vi "Check for Game Winner.vi"(8 "error in":errorcluster, 11 "Array - Numeric":dbl[][](array[numeric])) -> (0 "error out":errorcluster, 1 "Tie Game":bool, 2 "Player 1 wins":bool, 3 "Game Won":bool)   [LabVIEW 2021]
panel:
  out "Player 2 wins":bool
  out "diag subarray 2":dbl[](array[numeric])
  out "diag subarray 1":dbl[](array[numeric])
  out "col subarray 1":dbl[](array[numeric])
  out "col subarray 2":dbl[](array[numeric])
  out "col subarray 3":dbl[](array[numeric])
  out "row subarray 3":dbl[](array[numeric])
  out "row subarray 2":dbl[](array[numeric])
  out "row subarray 1":dbl[](array[numeric])
  # "Check rows\nCheck columns\nCheck diagonal 1 (top left to bot right)\nCheck diagonal 2 (bot left to top right)"
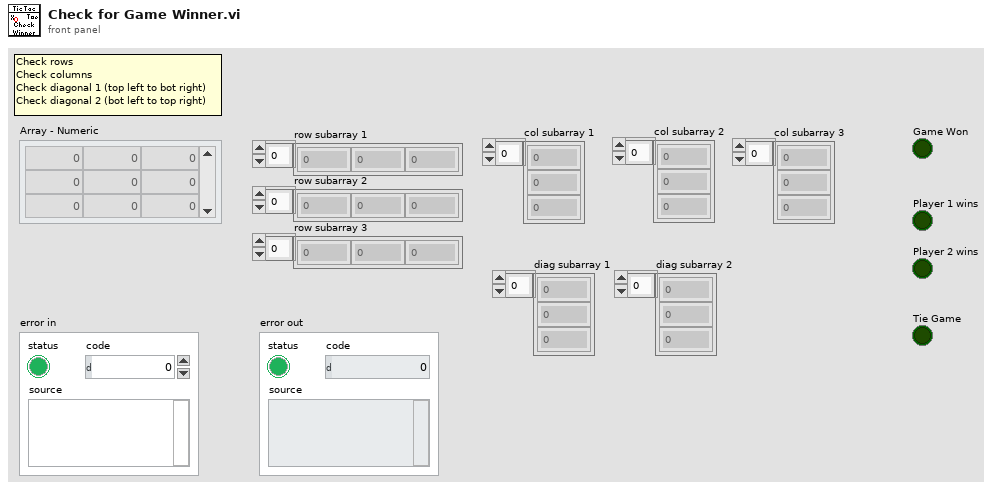
[diagram p1: front panel]
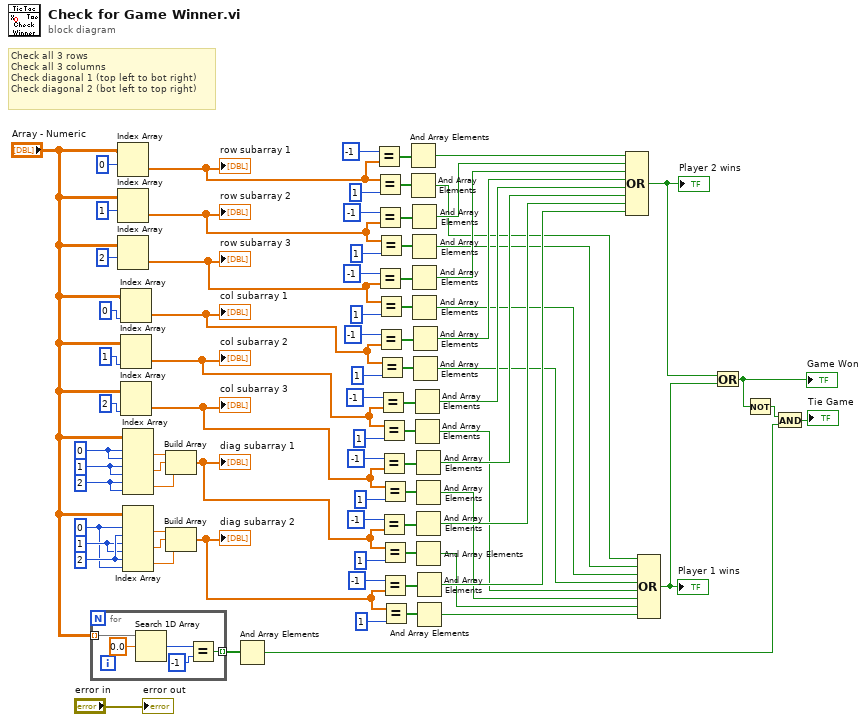
[diagram p0: block diagram]
diagram:
  w68 = 2 ("index (row)")
  w67 = 1 ("index (row)")
  w66 = 0 ("index (row)")
  w75 = 2 ("index (row)")
  w76 = 1 ("index (row)")
  w77 = 0 ("index (row)")
  # "Check all 3 rows\nCheck all 3 columns\nCheck diagonal 1 (top left to bot right)\nCheck diagonal 2 (bot left to top right)"
  n1 = for {
    tunnel: "Array - Numeric" -> [w88] mode=indexing
    tunnel: [w84] -> w5 mode=indexing
    n2 = Search 1D Array(1D array=w88, element=0.0) -> (index of element=w86:i32)  [unwired: 1 in]
    n3 = Equal?(x=w86, y=-1 ("index (row)")) -> (x = y?=w84:bool)
  }
  n4 = Index Array(array="Array - Numeric", index (row)=0) -> (element=w63:dbl[])  [unwired: 1 in]
  "row subarray 1" <- w63
  n5 = Index Array(array="Array - Numeric", index (row)=1) -> (element=w48:dbl[])  [unwired: 1 in]
  "row subarray 2" <- w48
  n6 = Index Array(array="Array - Numeric", index (row)=2) -> (element=w47:dbl[])  [unwired: 1 in]
  "row subarray 3" <- w47
  n7 = Index Array(array="Array - Numeric", index (col)=0 ("index (row)")) -> (element=w46:dbl[])  [unwired: 1 in]
  "col subarray 1" <- w46
  n8 = Index Array(array="Array - Numeric", index (col)=1 ("index (row)")) -> (element=w29:dbl[])  [unwired: 1 in]
  "col subarray 2" <- w29
  n9 = Index Array(array="Array - Numeric", index (col)=2 ("index (row)")) -> (element=w28:dbl[])  [unwired: 1 in]
  "col subarray 3" <- w28
  n10 = Index Array(array="Array - Numeric", index (row) #1=w77, index (col) #1=w77, index (row) #2=w76, index (col) #2=w76, index (row) #3=w75, index (col) #3=w75) -> (element #1=w74:dbl, element #2=w73:dbl, element #3=w72:dbl)
  n11 = Index Array(array="Array - Numeric", index (row) #1=w66, index (col) #1=w68, index (row) #2=w67, index (col) #2=w67, index (row) #3=w68, index (col) #3=w66) -> (element #1=w69:dbl, element #2=w70:dbl, element #3=w71:dbl)
  n12 = Build Array(w74, w73, w72) -> (w27:dbl[])
  "diag subarray 1" <- w27
  n13 = Build Array(w69, w70, w71) -> (w26:dbl[])
  "diag subarray 2" <- w26
  n14 = And Array Elements(Boolean array=w5) -> (logical AND=w2:bool)
  n15 = Equal?(x=-1 ("index (row)"), y=w63) -> (x = y?=w62:bool[])
  n16 = Equal?(x=w63, y=1 ("index (row)")) -> (x = y?=w61:bool[])
  n17 = Equal?(x=-1 ("index (row)"), y=w48) -> (x = y?=w59:bool[])
  n18 = Equal?(x=-1 ("index (row)"), y=w47) -> (x = y?=w51:bool[])
  n19 = Equal?(x=w48, y=1 ("index (row)")) -> (x = y?=w60:bool[])
  n20 = Equal?(x=w47, y=1 ("index (row)")) -> (x = y?=w52:bool[])
  n21 = Equal?(x=-1 ("index (row)"), y=w46) -> (x = y?=w54:bool[])
  n22 = Equal?(x=w46, y=1 ("index (row)")) -> (x = y?=w53:bool[])
  n23 = Equal?(x=-1 ("index (row)"), y=w29) -> (x = y?=w32:bool[])
  n24 = Equal?(x=w29, y=1 ("index (row)")) -> (x = y?=w33:bool[])
  n25 = Equal?(x=-1 ("index (row)"), y=w28) -> (x = y?=w35:bool[])
  n26 = Equal?(x=-1 ("index (row)"), y=w27) -> (x = y?=w43:bool[])
  n27 = Equal?(x=w28, y=1 ("index (row)")) -> (x = y?=w34:bool[])
  n28 = Equal?(x=w27, y=1 ("index (row)")) -> (x = y?=w42:bool[])
  n29 = Equal?(x=-1 ("index (row)"), y=w26) -> (x = y?=w40:bool[])
  n30 = Equal?(x=w26, y=1 ("index (row)")) -> (x = y?=w41:bool[])
  n31 = And Array Elements(Boolean array=w62) -> (logical AND=w25:bool)
  n32 = And Array Elements(Boolean array=w61) -> (logical AND=w10:bool)
  n33 = And Array Elements(Boolean array=w59) -> (logical AND=w24:bool)
  n34 = And Array Elements(Boolean array=w60) -> (logical AND=w11:bool)
  n35 = And Array Elements(Boolean array=w51) -> (logical AND=w23:bool)
  n36 = And Array Elements(Boolean array=w52) -> (logical AND=w12:bool)
  n37 = And Array Elements(Boolean array=w54) -> (logical AND=w22:bool)
  n38 = And Array Elements(Boolean array=w53) -> (logical AND=w13:bool)
  n39 = And Array Elements(Boolean array=w32) -> (logical AND=w21:bool)
  n40 = And Array Elements(Boolean array=w33) -> (logical AND=w14:bool)
  n41 = And Array Elements(Boolean array=w35) -> (logical AND=w20:bool)
  n42 = And Array Elements(Boolean array=w34) -> (logical AND=w15:bool)
  n43 = And Array Elements(Boolean array=w43) -> (logical AND=w19:bool)
  n44 = And Array Elements(Boolean array=w42) -> (logical AND=w16:bool)
  n45 = And Array Elements(Boolean array=w40) -> (logical AND=w18:bool)
  n46 = And Array Elements(Boolean array=w41) -> (logical AND=w17:bool)
  n47 = Compound Arithmetic op=OR(w25, w24, w23, w22, w21, w20, w19, w18) -> (w8:bool)
  "Player 2 wins" <- w8
  n48 = Compound Arithmetic op=OR(w10, w11, w12, w13, w14, w15, w16, w17) -> (w9:bool)
  "Player 1 wins" <- w9
  n49 = Or(x=w8, y=w9) -> (x .or. y?=w4:bool)
  "Game Won" <- w4
  n50 = Not(x=w4) -> (.not. x?=w3:bool)
  n51 = And(x=w3, y=w2) -> (x .and. y?=→"Tie Game":bool)
  "error out" <- "error in"
